vi "Delete Macro.vi"(7 "Macro Name":string, 8 "error in (no error)":errorcluster, 11 "App Data Directory":path) -> (0 "error out":errorcluster)   [LabVIEW 2020, in "MacroAssert.lvlib"]
doc: "Deletes the INI associated with <B>Macro Name</B> from <B>App Data Directory</B>."
uses:
  MacroAssert.lvlib
  <userlib>/_OpenG.lib/file/file.llb/openg_file.lvlib
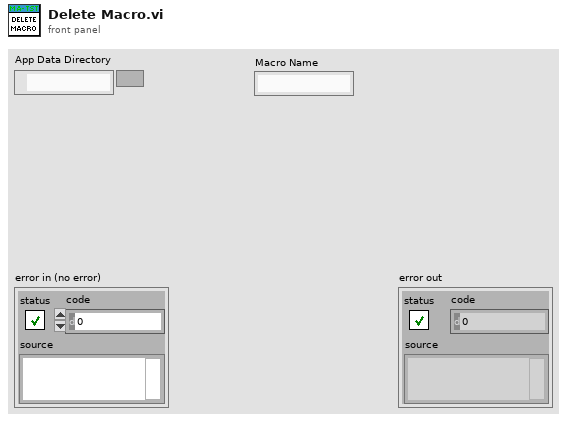
[diagram p1: front panel]
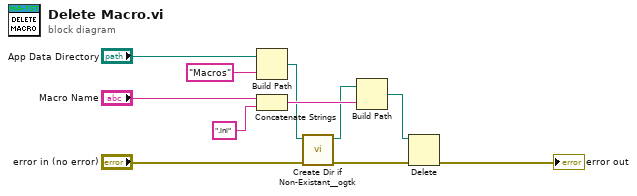
[diagram p0: block diagram]
diagram:
  n1 = Build Path(base path="App Data Directory", name or relative path="Macros" ("string")) -> (appended path=w3:path)
  n2 = Concatenate Strings("Macro Name", ".ini" ("string")) -> (w9:string)
  n3 = call <userlib>:"Create Dir if Non-Existant__ogtk.vi"("error in (no error)"="error in (no error)", "Directory Path"=w3) -> ("error out"=w4:errorcluster, "dup Directory Path"=w2:path)  [unwired: 7 in, 1 out]
  n4 = Build Path(base path=w2, name or relative path=w9) -> (appended path=w7:path)
  n5 = Delete(path (use dialog)=w7, error in=w4) -> (error out=→"error out":errorcluster)  [unwired: 3 in, 2 out]
